vi "get_calibration.vi"(6 "timeout (25000ms)":i32=25000, 8 "error in (no error)":errorcluster, 10 "Calibration":T1[](array[typedef]), 11 "daemon reference in":refnum<k5>) -> (0 "error out":errorcluster, 1 "response":string, 2 "values":dbl[](array[numeric]) format="%_6g", 3 "daemon reference out":refnum<k5>, 5 "command out":string="random")   [LabVIEW 2017]
doc: "<b>Command: </b>\"get_calibration\"\n\n<b>Description: </b> Instructs the target to return the specified calibration parameter values.\n\n<b>Parameters: </b> \n\n 1. Parameter Array [max 20]\n____________________________________________\nDIPC 692 Daemon API 10.0.0.1\nSam Tee - Dyson Technology Ltd\nCopyright (c) 2024, Dyson Technology Ltd"
uses:
  typdef/calibration.ctl
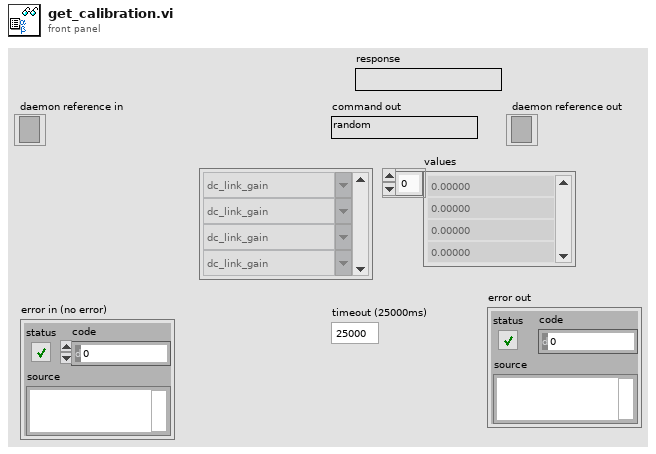
[diagram p1: front panel]
types:
  T1 = typedef "calibration.ctl" = string
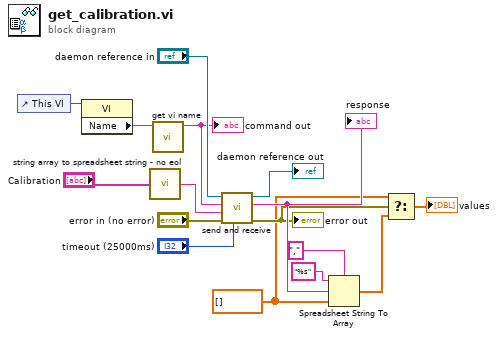
[diagram p0: block diagram]
diagram:
  w4 = dbl[] []
  n1 = control-ref of="This VI"() -> (w12:refnum<vi>)
  n2 = property class="VI"(reference=w12) -> ("Name"=w11:string)  [unwired: 1 in, 2 out]
  n3 = call "string array to spreadsheet string - no eol.vi"("string array"="Calibration") -> ("spreadsheet string - no eol"=w6:string)
  n4 = call "get vi name.vi"("library.lvlib:name.vi"=w11) -> ("vi name"=w10:string)  [unwired: 10 in]
  "command out" <- w10
  n5 = call "send and receive.vi"("timeout (25000ms)"="timeout (25000ms)", "error in (no error)"="error in (no error)", "data"=w6, "command"=w10, "daemon reference in"="daemon reference in") -> ("error out"=w5:errorcluster, "response"=w9:string, "daemon reference out"=→"daemon reference out":refnum<k5>)  [unwired: 4 in]
  "error out" <- w5
  "response" <- w9
  n6 = Spreadsheet String To Array(delimiter (Tab)=",", format string="%s", spreadsheet string=w9, array type (2D Dbl)=w4) -> (array=w3:dbl[])
  n7 = Select(t=w4, s=w5, f=w3) -> (s? t:f=→"values":dbl[])
